vi "VSS_GoTo.vi"(10 "SetPoint":dbl[](array[numeric])=[100.0, 100.0, 0.0], 11 "Position":dbl[](array[numeric])=[208.6539306640625, -200.4281768798828, 3.141592653589793]) -> (3 "Output Vel":dbl[](array[numeric])=[0.0, 0.0, 0.8321627905647668])   [LabVIEW 2018]
uses:
  <vilib>/Analysis/coordinate.llb/Wrap Angle (scalar).vi
  <vilib>/Analysis/_algsub.llb/Real Vector Norm.vi
  <vilib>/Analysis/NI_AAL_Angle.lvlib
  <vilib>/Analysis/NI_AALPro.lvlib
panel:
  out "Angular":dbl(graph)=0.8321627905647668
  in  "fc angular":dbl=80.0
  out "Tangent":dbl(graph)
  in  "fc tangent":dbl=0.85
  out "NaN":bool
  in  "y 2":dbl=20.0 format="%#_13g"
  in  "y":dbl=0.4 format="%#_13g"
  in  "Limits tangent":cluster{"output high":dbl, "output low":dbl}={"output high"=1.2, "output low"=-1.2}
  in  "PID gains tangent":T1={"proportional gain (Kc)"=0.0044, "integral time (Ti, min)"=0.0, "derivative time (Td, min)"=-0.085}
  in  "Limits ang":cluster{"output high":dbl, "output low":dbl}={"output high"=1.0, "output low"=-1.0}
  in  "PID gains ang":T1={"proportional gain (Kc)"=0.5, "integral time (Ti, min)"=0.0, "derivative time (Td, min)"=-0.08}
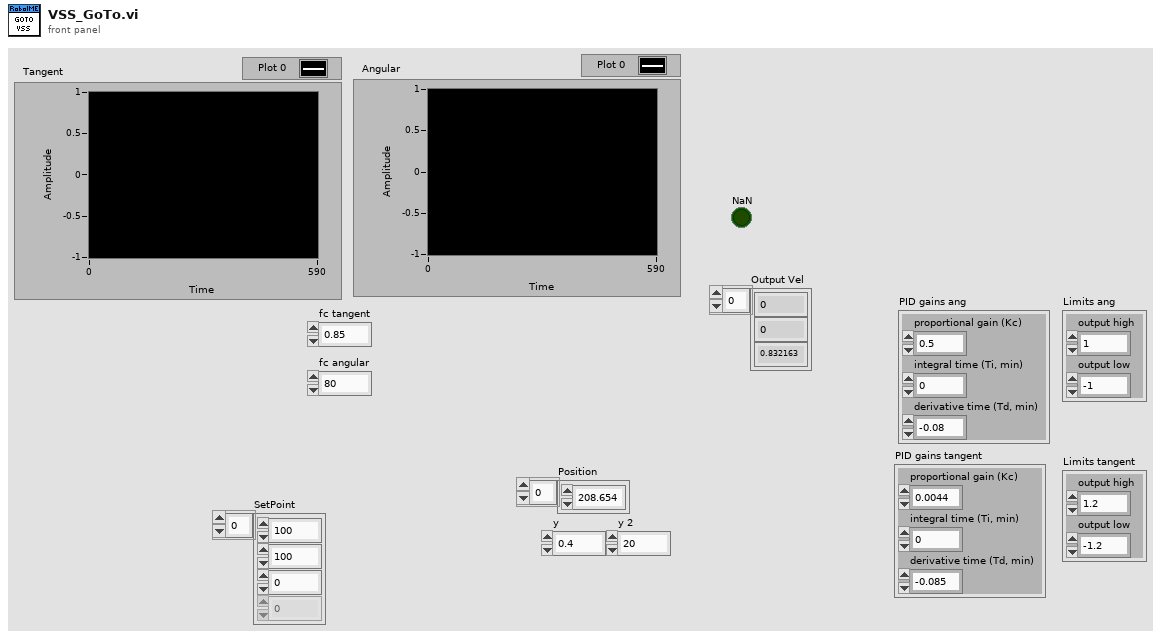
[diagram p1: front panel]
types:
  T1 = cluster{"proportional gain (Kc)":dbl, "integral time (Ti, min)":dbl, "derivative time (Td, min)":dbl}
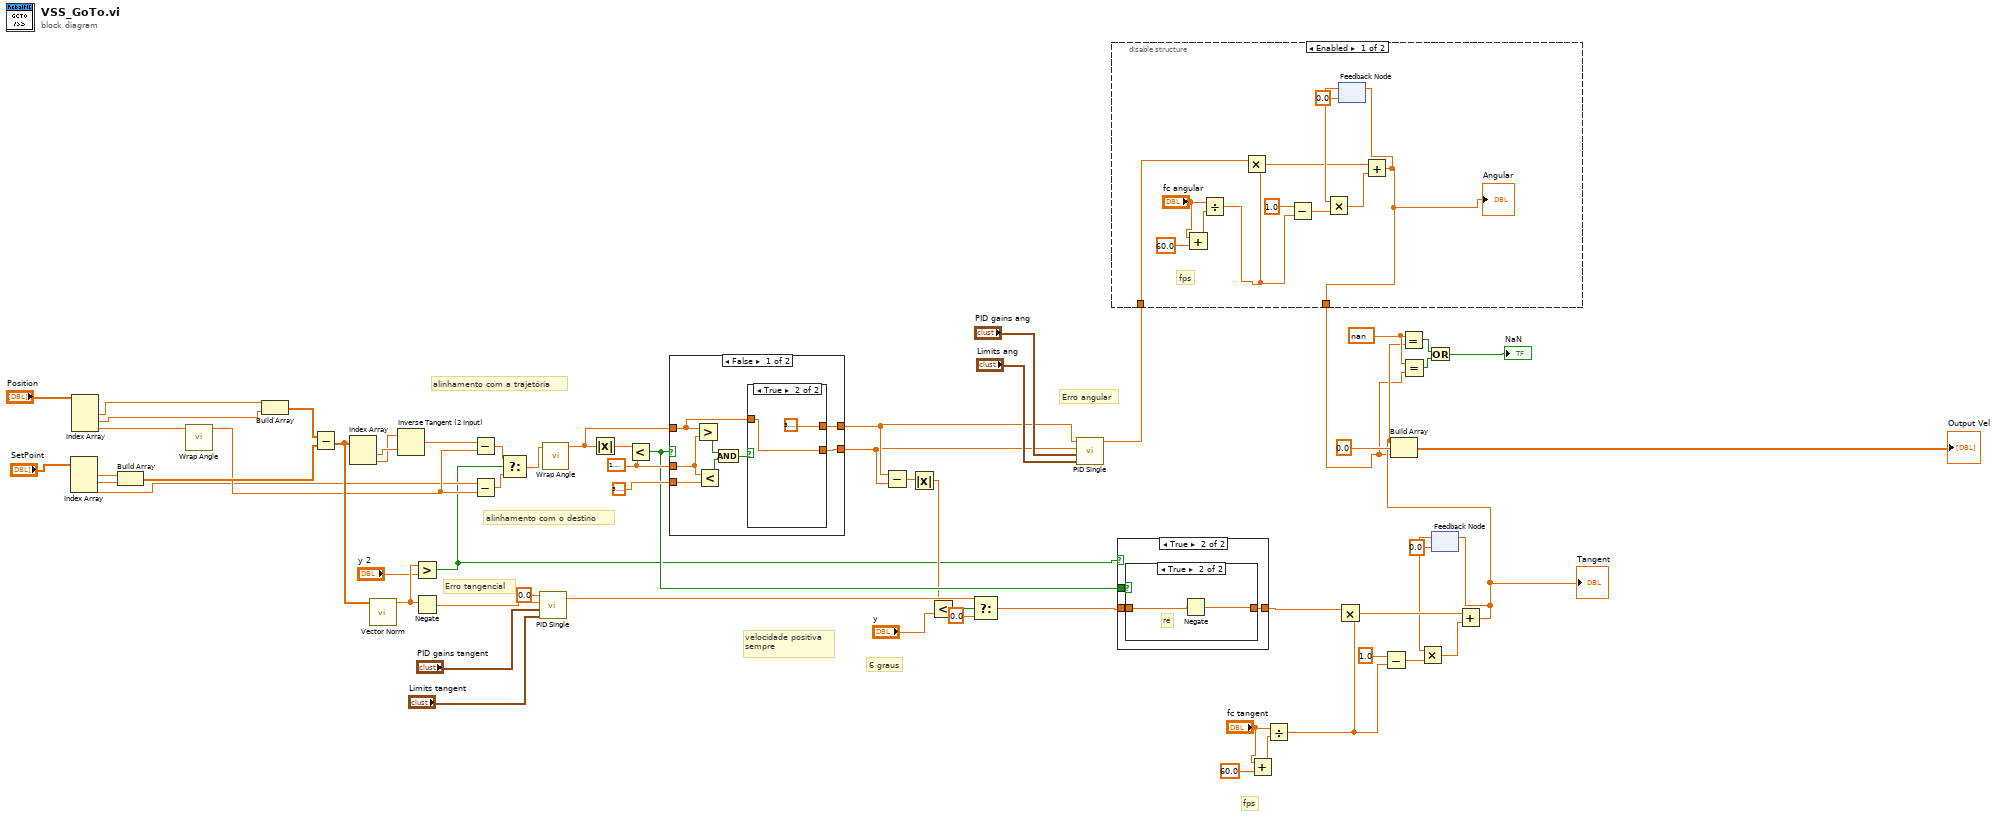
[diagram p0: block diagram]
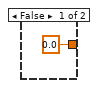
[diagram p3: hidden frame]
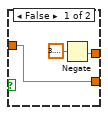
[diagram p5: hidden frame]
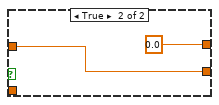
[diagram p6: hidden frame]
diagram:
  w19 = nan
  w40 = 1.5707963267948966
  # "fps"
  # "alinhamento com o destino"
  # "alinhamento com a trajetória"
  # "velocidade positiva\nsempre"
  # "Erro tangencial"
  # "Erro angular"
  # "6 graus"
  n1 = Index Array(array="SetPoint") -> (element #1=w47:dbl, element #2=w46:dbl, element #3=w28:dbl)  [unwired: 3 in]
  n2 = Index Array(array="Position") -> (element #1=w50:dbl, element #2=w49:dbl, element #3=w42:dbl)  [unwired: 3 in]
  n3 = Build Array(w47, w46) -> (w45:dbl[])
  n4 = call-poly <vilib>:"Wrap Angle.vi"("angle in"=w42) -> ("angle out"=w29:dbl)  [unwired: 9 in, 1 out]
  n5 = Build Array(w50, w49) -> (w60:dbl[])
  n6 = Subtract(x=w60, y=w45) -> (x-y=w31:dbl[])
  n7 = Index Array(array=w31) -> (element #1=w59:dbl, element #2=w58:dbl)  [unwired: 2 in]
  n8 = call-poly <vilib>:"Vector Norm.vi"("Input Vector"=w31) -> ("norm"=w24:dbl)  [unwired: 9 in, 1 out]
  n9 = Inverse Tangent (2 Input)(1:w59, 2:w58) -> (0:w30:dbl)
  n10 = Greater?(x=w24, y="y 2") -> (0:w21:bool)
  n11 = Negate(x=w24) -> (-x=w35:dbl)
  n12 = Subtract(x=w30, y=w29) -> (x-y=w26:dbl)
  n13 = Subtract(x=w28, y=w29) -> (x-y=w25:dbl)
  n14 = Select(t=w26, s=w21, f=w25) -> (s? t:f=w27:dbl)
  n15 = call "PID Single.vi"("Limits"="Limits tangent", "PID gains in"="PID gains tangent", "Variable"=w35, "Setpoint"=0.0) -> ("Out"=w52:dbl)  [unwired: 7 in]
  n16 = call-poly <vilib>:"Wrap Angle.vi"("angle in"=w27) -> ("angle out"=w38:dbl)  [unwired: 9 in, 1 out]
  n17 = Absolute Value(x=w38) -> (abs(x)=w41:dbl)
  n18 = Less?(x=w41, y=w40) -> (x < y?=w36:bool)
  n19 = case shown="False" w36 {
    tunnel: w38 -> [w62 w76]
    tunnel: [w63 w76] -> w33
    tunnel: w40 -> [w69 _]
    tunnel: 3.141592653589793 -> [w68 _]
    tunnel: [w64 0.0 ("Variable")] -> w34
    frame False {
      n20 = Greater?(x=w62, y=w69) -> (0:w66:bool)
      n21 = Less?(x=w69, y=w68) -> (x < y?=w67:bool)
      n22 = And(x=w66, y=w67) -> (x .and. y?=w65:bool)
      n23 = case shown="True" w65 {
        tunnel: [w72 3.141592653589793] -> w64
        tunnel: [w70 w73] -> w63
        tunnel: w62 -> [w70 w73]
        frame False {
          n24 = Negate(x=3.141592653589793) -> (-x=w72:dbl)
        }
        frame True {
        }
      }
    }
    frame True {
    }
  }
  n25 = Subtract(x=w34, y=w33) -> (x-y=w32:dbl)
  n26 = Absolute Value(x=w32) -> (abs(x)=w22:dbl)
  n27 = Less?(x=w22, y="y") -> (x < y?=w53:bool)
  n28 = Select(t=w52, s=w53, f=0.0) -> (s? t:f=w37:dbl)
  n29 = call "PID Single.vi"("Limits"="Limits ang", "PID gains in"="PID gains ang", "Variable"=w33, "Setpoint"=w34) -> ("Out"=w2:dbl)  [unwired: 7 in]
  n30 = disable-structure shown="Enabled" {
    disable-tunnel: [w78 w89] -> w3
    disable-tunnel: w2 -> [w77 w89]
    frame Enabled {
      # "fps"
      n31 = Add(x="fc angular", y=60.0) -> (x+y=w82:dbl)
      n32 = Divide(x="fc angular", y=w82) -> (x/y=w79:dbl)
      n33 = Multiply(x=w77, y=w79) -> (x*y=w83:dbl)
      n34 = Subtract(x=1.0, y=w79) -> (x-y=w85:dbl)
      n35 = feedback #1(0.0) -> (w86:dbl)
      n36 = Multiply(x=w86, y=w85) -> (x*y=w87:dbl)
      n37 = Add(x=w83, y=w87) -> (x+y=w78:dbl)
      "Angular" <- w78
      n38 = feedback-in #1(w78) -> ()
    }
    frame Disabled {
    }
  }
  n39 = case shown="True" w21 {
    tunnel: w37 -> [_ w93]
    tunnel: w36 -> [_ w92]
    tunnel: [0.0 ("f") w91] -> w15
    frame False {
    }
    frame True {
      n40 = case shown="True" w92 {
        tunnel: w93 -> [w94 w96]
        tunnel: [w94 w95] -> w91
        frame False {
        }
        frame True {
          # "ré"
          n41 = Negate(x=w96) -> (-x=w95:dbl)
        }
      }
    }
  }
  n42 = Add(x="fc tangent", y=60.0) -> (x+y=w5:dbl)
  n43 = Divide(x="fc tangent", y=w5) -> (x/y=w8:dbl)
  n44 = Multiply(x=w15, y=w8) -> (x*y=w14:dbl)
  n45 = Subtract(x=1.0, y=w8) -> (x-y=w12:dbl)
  n46 = Equal?(x=w19, y=w3) -> (x = y?=w18:bool)
  n47 = feedback #2(0.0) -> (w11:dbl)
  n48 = Multiply(x=w11, y=w12) -> (x*y=w10:dbl)
  n49 = Add(x=w14, y=w10) -> (x+y=w4:dbl)
  "Tangent" <- w4
  n50 = Build Array(w4, 0.0 ("element"), w3) -> (→"Output Vel":dbl[])
  n51 = Equal?(x=w19, y=w4) -> (x = y?=w17:bool)
  n52 = Or(x=w17, y=w18) -> (x .or. y?=→"NaN":bool)
  n53 = feedback-in #2(w4) -> ()
